vi "ViewStringMessageOnMainScreen.vi"(7 "Criticity":T1, 8 "error in (no error)":errorcluster, 11 "Message":string) -> (0 "error out":errorcluster)   [LabVIEW 2009]
uses:
  030 - EVENTS/03 - ToMessageHandlerProcess/enumMessageCriticity.ctl
  030 - EVENTS/EnumFgvEventCommand.ctl
  030 - EVENTS/01 - ToHmiScheduler/ToHmiScheduler.ctl
  030 - EVENTS/01 - ToHmiScheduler/ToHmiSchedulerCommand.ctl
  030 - EVENTS/03 - ToMessageHandlerProcess/ToMessageHandlerEvent.ctl
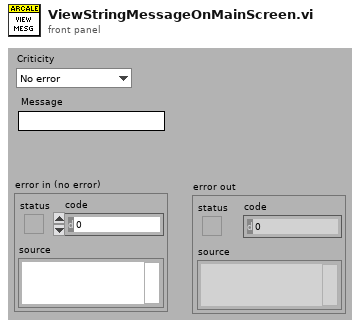
[diagram p1: front panel]
types:
  T1 = typedef "enumMessageCriticity.ctl" = enum16{"No error", "Info", "Warning", "Error", "Fatal error"}
  T2 = typedef "ToMessageHandlerEvent.ctl" = cluster{"date / time":timestamp, "Criticity":T1, "Emitter":string, "Message":string}
  T3 = typedef "ToHmiSchedulerCommand.ctl" = enum16{"Load screen", "Lock screen", "Unlock screen", "Close enable", "Close disable", "Start automatic progress bar", "Stop automatic progress bar", "Set progress bar value (0..100)", "Load previous screen", "Close application", "View message", "Clear message"}
  T4 = typedef "ToHmiScheduler.ctl" = cluster{"Command":T3, "Screen path":path, "Progress bar value":u8, "Screen Title":string, "To message handler event":T2}
  T5 = typedef "EnumFgvEventCommand.ctl" = enum16{"Setup", "Cleanup", "Get"}
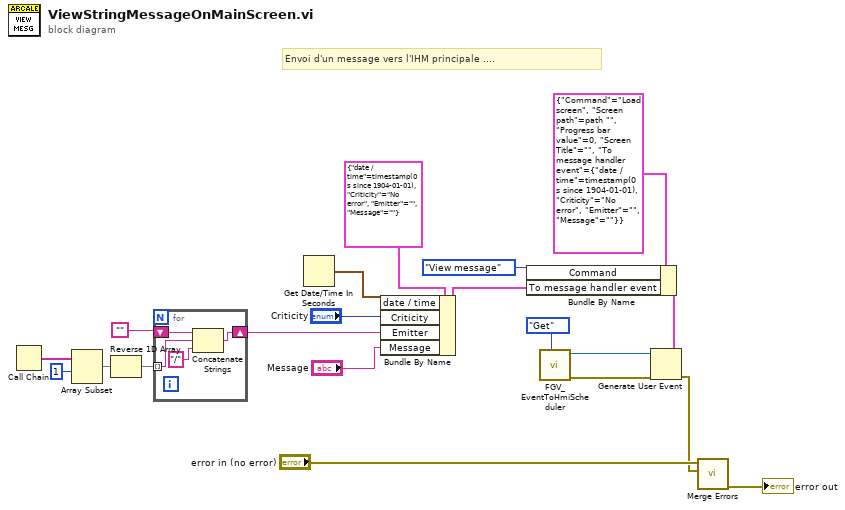
[diagram p0: block diagram]
diagram:
  # "Envoi d'un message vers l'IHM principale ...."
  n1 = Call Chain() -> (call chain=w5:string[])
  n2 = Array Subset(array=w5, index=1) -> (w7:string[])  [unwired: 1 in]
  n3 = Reverse 1D Array(array=w7) -> (reversed array=w9:string[])
  n4 = for {
    tunnel: w9 -> [w22] mode=indexing
    shift-right: [w24] -> w4
    shift-left: "" -> [w23]
    n5 = Concatenate Strings(w23, w22, "/" ("string")) -> (w24:string)
  }
  n6 = Get Date/Time In Seconds() -> (seconds since 1Jan1904=w2:timestamp)
  n7 = Bundle By Name(cluster=T2 {"date / time"=timestamp(0 s since 1904-01-01), "Criticity"=enum."No error", "Emitter"="", "Message"=""} ("To message handler event"), "date / time"=w2, "Criticity"="Criticity", "Emitter"=w4, "Message"="Message") -> (w10:T2)
  n8 = Bundle By Name(cluster=T4 {"Command"=enum."Load screen", "Screen path"=path "", "Progress bar value"=0, "Screen Title"="", "To message handler event"={"date / time"=timestamp(0 s since 1904-01-01), "Criticity"=enum."No error", "Emitter"="", "Message"=""}} ("event data"), "Command"=ToHmiSchedulerCommand."View message", "To message handler event"=w10) -> (w16:T4)
  n9 = call "FGV_EventToHmiScheduler.vi"("Command"=EnumFgvEventCommand."Get") -> ("error out"=w19:errorcluster, "ToHmiSchedulerEvent"=w18:refnum<user-event>)  [unwired: 9 in]
  n10 = Generate User Event(user event=w18, event data cluster=w16, error in=w19) -> (error out=w14:errorcluster)  [unwired: 1 out]
  n11 = call <vilib>:"Merge Errors.vi"("error in 2 (no error)"=w14, "error in 1 (no error)"="error in (no error)") -> ("error out"=→"error out":errorcluster)  [unwired: 5 in]
